vi "Start Point on Target.vi"(7 "Point dent":string, 8 "error in":errorcluster, 11 "Study Actor in":refnum<class "Study Actor.lvclass">) -> (0 "error out":errorcluster, 3 "Study Actor out":refnum<class "Study Actor.lvclass">)   [LabVIEW 2024, in "Study Actor.lvlib" / "Study Actor.lvclass"]
uses:
  Study Actor.lvclass
  HAL/MSS Target Actor/IMSS Target Actor Messages/Start Point Msg/Start Point Msg.lvclass/Start Point Msg.ctl
  <vilib>/ActorFramework/Message Enqueuer/Message Enqueuer.lvclass/Message Enqueuer.ctl
  <vilib>/ActorFramework/Message Enqueuer/Enqueue.vi
  HAL/MSS Target Actor/IMSS Target Actor Messages/Start Point Msg/Start Point Msg.lvclass
  <vilib>/Utility/LVClass/Get LV Class Name.vi
  <resource>/AFDebug/Generate Trace for Message.vi
  <vilib>/ActorFramework/Message Priority Queue/Priority Enqueue.vi
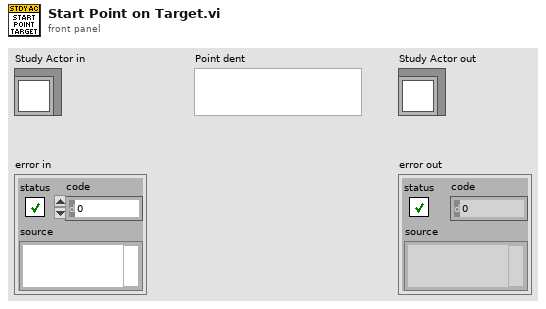
[diagram p1: front panel]
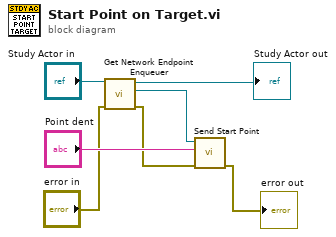
[diagram p0: block diagram]
diagram:
  n1 = call "Get Network Endpoint Enqueuer.vi"("error in"="error in", "Study Actor in"="Study Actor in") -> ("error out"=w1:errorcluster, "Network Endpoint Enqueuer"=w5:refnum<class "Message Enqueuer.lvclass">, "Study Actor out"=→"Study Actor out":refnum<class "Study Actor.lvclass">)  [unwired: 6 in, 1 out]
  n2 = call "Send Start Point.vi"("error in (no error)"=w1, "Point Ident"="Point dent", "Message Enqueuer"=w5) -> ("error out"=→"error out":errorcluster)  [unwired: 7 in, 1 out]
